vi "Keithley current indicator.vi"(8 "error in (no error)":errorcluster, 11 "VISA resource name":refnum<visa-resource-name>) -> (0 "error out":errorcluster, 2 "appended array":sgl[](array[numeric]), 3 "VISA resource name out":refnum<visa-resource-name>)   [LabVIEW 2017]
uses:
  <instrlib>/Keithley 24XX/Public/Data/Read (Single Point).vi
  <instrlib>/Keithley 24XX/Keithley 24XX.lvlib
panel:
  out "Waveform Chart":sgl[](graph)
  in  "stop":bool
  out "Current (A)":sgl
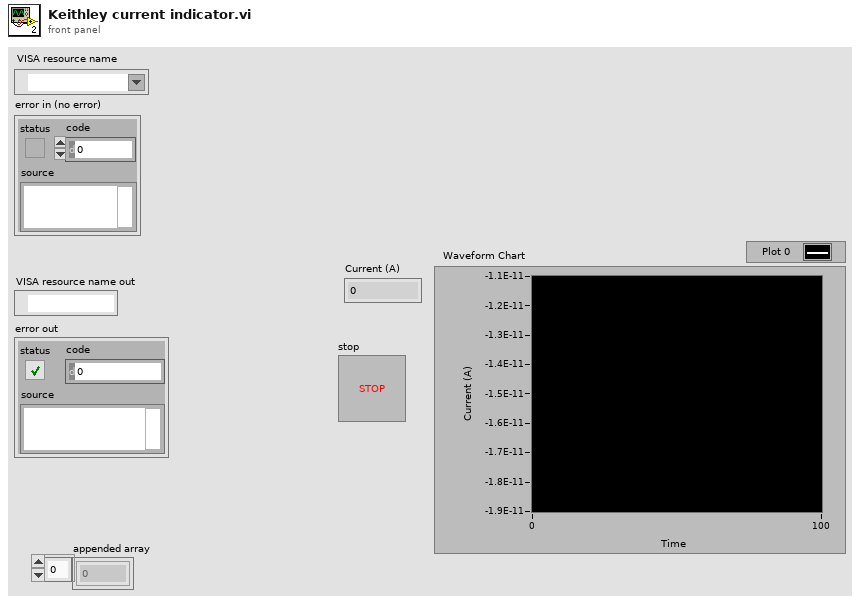
[diagram p1: front panel]
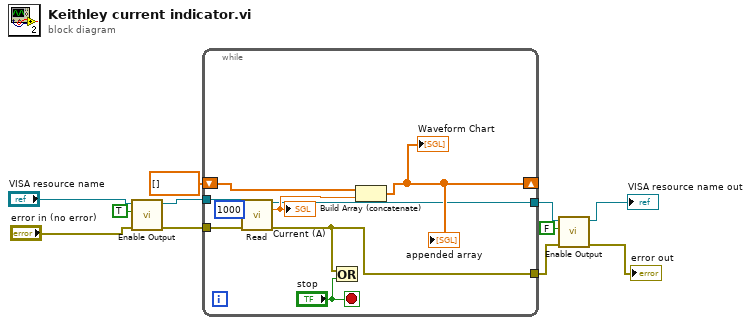
[diagram p0: block diagram]
diagram:
  n1 = call <instrlib>:"Enable Output.vi"("error in (no error)"="error in (no error)", "Enable Output (T: Enable)"=TRUE, "VISA resource name"="VISA resource name") -> ("error out"=w6:errorcluster, "VISA resource name out"=w7:refnum<visa-resource-name>)  [unwired: 7 in]
  n2 = while {
    tunnel: w7 -> [w20]
    tunnel: w6 -> [w19]
    shift-right: [w16] -> _
    shift-left: sgl[] [] -> [w18]
    tunnel: [w13] -> w4
    tunnel: [w12] -> w3
    stop <- "stop" stop-if-true
    n3 = call-poly <instrlib>:"Read.vi"("VISA resource name"=w20, "Timeout (10000 ms)"=1000, "error in (no error)"=w19) -> ("VISA resource name out"=w12:refnum<visa-resource-name>, "Current"=w17:sgl, "error out"=w13:errorcluster)  [unwired: 6 in, 4 out]
    "Current (A)" <- w17
    n4 = Or(x=w13, y="stop") -> ()  [unwired: 1 out]
    n5 = Build Array (concatenate)(w18, w17) -> (w16:sgl[])
    "Waveform Chart" <- w16
    "appended array" <- w16
  }
  n6 = call <instrlib>:"Enable Output.vi"("error in (no error)"=w4, "Enable Output (T: Enable)"=FALSE, "VISA resource name"=w3) -> ("error out"=→"error out":errorcluster, "VISA resource name out"=→"VISA resource name out":refnum<visa-resource-name>)  [unwired: 7 in]
